vi "10_loop.vi"(11 "文字列":string) -> (3 "検索文字列":string)   [LabVIEW 2019]
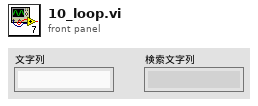
[diagram p1: front panel]
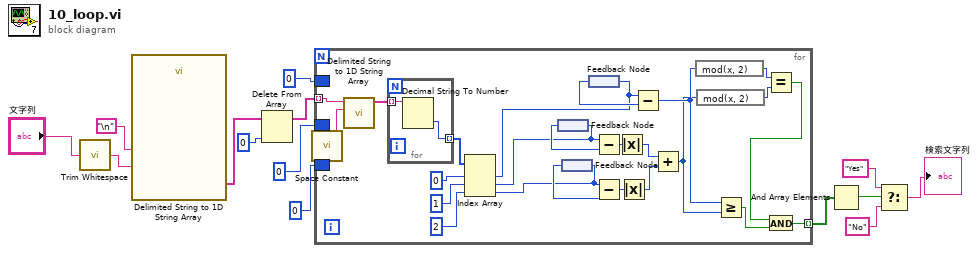
[diagram p0: block diagram]
diagram:
  n1 = call <vilib>:"Trim Whitespace.vi"("string"="文字列") -> ("trimmed string"=w1:string)  [unwired: 1 in]
  n2 = call <vilib>:"Delimited String to 1D String Array.vi"("delimiter"="\n", "delimited string"=w1) -> ("string array"=w5:string[])  [unwired: 9 in]
  n3 = Delete From Array ("配列から削除")(array=w5, index=0) -> (array with subset deleted=w6:string[])  [unwired: 1 in, 1 out]
  n4 = for {
    tunnel: w6 -> [w38] mode=indexing
    tunnel: [w20] -> w10 mode=indexing
    border: 0 -> [_]
    border: 0 -> [_]
    border: 0 -> [_]
    n5 = call <vilib>:"Space Constant.vi"() -> ("String"=w37:string)
    n6 = call <vilib>:"Delimited String to 1D String Array.vi"("delimiter"=w37, "delimited string"=w38) -> ("string array"=w36:string[])  [unwired: 9 in]
    n7 = for {
      tunnel: w36 -> [w40] mode=indexing
      tunnel: [w39] -> w34 mode=indexing
      n8 = Decimal String To Number(string=w40) -> (number=w39:i32)  [unwired: 2 in, 1 out]
    }
    n9 = Index Array ("指標配列")(array=w34, index #1=0, index #2=1, index #3=2) -> (element #1=w30:i32, element #2=w15:i32, element #3=w19:i32)
    n10 = feedback-in #1(w15) -> ()
    n11 = feedback #1() -> (w29:i32)
    n12 = feedback-in #2(w19) -> ()
    n13 = feedback #2() -> (w28:i32)
    n14 = feedback-in #3(w30) -> ()
    n15 = feedback #3() -> (w31:i32)
    n16 = Subtract(x=w15, y=w29) -> (x-y=w27:i32)
    n17 = Subtract(x=w19, y=w28) -> (x-y=w26:i32)
    n18 = Absolute Value(x=w27) -> (abs(x)=w18:i32)
    n19 = Absolute Value(x=w26) -> (abs(x)=w17:i32)
    n20 = Subtract(x=w30, y=w31) -> (x-y=w23:i32)
    n21 = Add(x=w18, y=w17) -> (x+y=w22:i32)
    n22 = expression code="mod(x, 2)"(w23) -> (w25:i32)
    n23 = expression code="mod(x, 2)"(w22) -> (w24:i32)
    n24 = Greater Or Equal?(x=w23, y=w22) -> (x >= y?=w21:bool)
    n25 = Equal?(x=w25, y=w24) -> (x = y?=w16:bool)
    n26 = And(x=w16, y=w21) -> (x .and. y?=w20:bool)
  }
  n27 = And Array Elements(Boolean array=w10) -> (logical AND=w13:bool)
  n28 = Select(t="Yes" ("検索文字列"), s=w13, f="No" ("検索文字列")) -> (s? t:f=→"検索文字列":string)
